vi "Tester.vi"() -> ()   [LabVIEW 2017]
uses:
  Filled Text Fields Actor/Filled Text Fields Facade.ctl
  Filled Text Fields Actor/Filled Text Fields/Get Value Change Event.vi
  Filled Text Fields Actor/Filled Text Fields/Set Value.vi
  Filled Text Fields Actor/Filled Text Fields/Set Animate.vi
  Filled Text Fields Actor/Filled Text Fields/Get Theme Font.vi
  Filled Text Fields Actor/Filled Text Fields/Set Theme Font.vi
  Filled Text Fields Actor/Filled Text Fields/Set Helper Text.vi
  Filled Text Fields Actor/Filled Text Fields/Filled Text Fields.lvclass
  Filled Text Fields Actor/Filled Text Fields.lvlib
panel:
  out "Data":string
  in  "Help text":string
  in  "Password Display":bool
  in  "Animate":bool
  in  "Apply":bool
  in  "String":string
  in  "Filled Text Fields":T1 caption="Filled String"
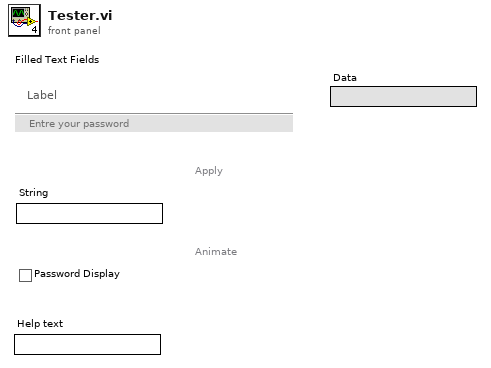
[diagram p1: front panel]
types:
  T1 = typedef "Filled Text Fields.lvlib/Filled Text Fields Facade.ctl" = cluster{"Label":string}
  T2 = typedef "Theme.lvlib/Theme.Font.lvclass/Font.ctl" = cluster{"Size":u32, "Shrink Size":u32, "Name":string, "Password Display":bool}
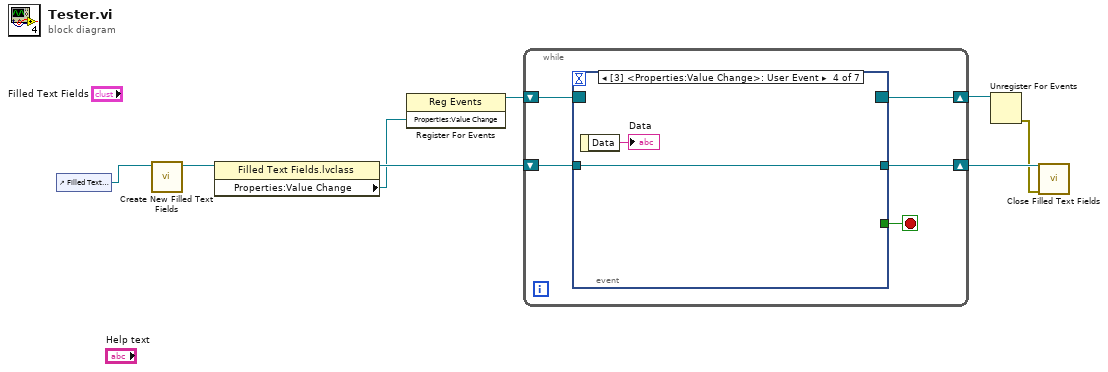
[diagram p0: block diagram]
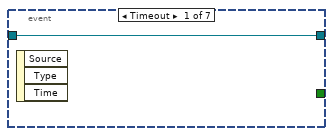
[diagram p2: hidden frame]
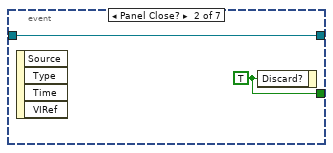
[diagram p3: hidden frame]
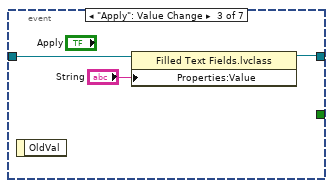
[diagram p4: hidden frame]
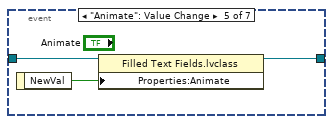
[diagram p5: hidden frame]
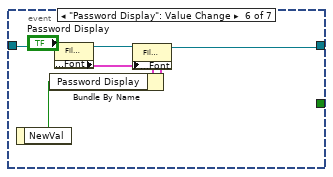
[diagram p6: hidden frame]
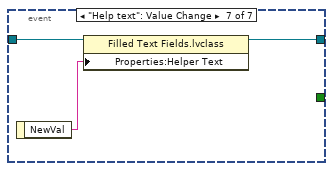
[diagram p7: hidden frame]
diagram:
  n1 = control-ref of="Filled Text Fields"() -> (w7:refnum<vi>)
  n2 = call "Create New Filled Text Fields.vi"("Filled Text Fields Ref"=w7) -> ("Filled Text Fields out"=w8:refnum<class "Filled Text Fields.lvclass">)  [unwired: 9 in, 1 out]
  n3 = property class="Filled Text Fields.lvclass"(reference=w8) -> (reference out=w6:refnum<class "Filled Text Fields.lvclass">, "Properties:Value Change"=w5:refnum<user-event>)  [unwired: 1 in, 1 out]
  n4 = register-events(w5) -> (reference out=w4:refnum<event-registration>)  [unwired: 2 in, 1 out]
  n5 = while {
    shift-right: [w10] -> w3
    shift-left: w4 -> [w11]
    shift-right: [w9] -> w2
    shift-left: w6 -> [w12]
    stop <- w13 stop-if-true
    n6 = event shown="[3] <Properties:Value Change>: User Event" {
      selector: w11 -> [_ _ _ _ _ _ _]
      dyn-events: [_ _ _ _ _ _ _] -> w10
      timeout: _ -> [_ _ _ _ _ _ _]
      tunnel: [_ w16 _ _ _ _ _] -> w13
      tunnel: w12 -> [w14 w15 w19 w21 w24 w30 w33]
      tunnel: [w14 w15 w17 w21 w22 w25 w31] -> w9
      event Timeout {
        n7 = event-data() -> ()  [unwired: 1 in, 3 out]
      }
      event Panel Close? {
        w16 = TRUE ("Discard?")
        n8 = event-data() -> ()  [unwired: 1 in, 4 out]
        n9 = event-data("Discard?"=w16) -> ()  [unwired: 1 in, 1 out]
      }
      event "Apply": Value Change {
        n10 = event-data() -> ()  [unwired: 1 in, 1 out]
        n11 = property class="Filled Text Fields.lvclass"(reference=w19, "Properties:Value"="String") -> (reference out=w17:refnum<class "Filled Text Fields.lvclass">)  [unwired: 1 in, 1 out]
      }
      event User Event {
        n12 = event-data() -> ("Data"=→"Data":string)  [unwired: 1 in]
      }
      event "Animate": Value Change {
        n13 = event-data() -> ("NewVal"=w23:bool)  [unwired: 1 in]
        n14 = property class="Filled Text Fields.lvclass"(reference=w24, "Properties:Animate"=w23) -> (reference out=w22:refnum<class "Filled Text Fields.lvclass">)  [unwired: 1 in, 1 out]
      }
      event "Password Display": Value Change {
        n15 = event-data() -> ("NewVal"=w26:bool)  [unwired: 1 in]
        n16 = property class="Filled Text Fields.lvclass"(reference=w30) -> (reference out=w29:refnum<class "Filled Text Fields.lvclass">, "Properties:Font"=w28:T2)  [unwired: 1 in, 1 out]
        n17 = Bundle By Name(cluster=w28, "Password Display"=w26) -> (w27:T2)
        n18 = property class="Filled Text Fields.lvclass"(reference=w29, "Properties:Font"=w27) -> (reference out=w25:refnum<class "Filled Text Fields.lvclass">)  [unwired: 1 in, 1 out]
      }
      event "Help text": Value Change {
        n19 = event-data() -> ("NewVal"=w32:string)  [unwired: 1 in]
        n20 = property class="Filled Text Fields.lvclass"(reference=w33, "Properties:Helper Text"=w32) -> (reference out=w31:refnum<class "Filled Text Fields.lvclass">)  [unwired: 1 in, 1 out]
      }
    }
  }
  n21 = Unregister For Events(event registration refnum=w3) -> (error out=w1:errorcluster)  [unwired: 1 in]
  n22 = call "Close Filled Text Fields.vi"("error in (no error)"=w1, "Filled Text Fields in"=w2) -> ()  [unwired: 9 in, 1 out]
